vi "Get Section Indentation Length.vi"(10 "sections":string[](array[string]), 11 "info data":string) -> (3 "Indentation length":i32)   [LabVIEW 2013, in "infolib.lvlib"]
doc: "Checks if sections structure exists, if so divides string before the end of least significant section."
uses:
  infolib.lvlib
  <vilib>/regexp/Match Regular Expression.xnode
panel:
  out "submatch 1":string
  out "regexp":string
  # "testing string: (put \"1\" and \"2\" into section names)"
  # "blfdablad\n#startsection:: 1\njfkdla\n#startsection:: 2\ngroup2group2\n\t  \t#endsection:: 2\njdfkls\n#endsection:: 1\njfdklajfkdl"
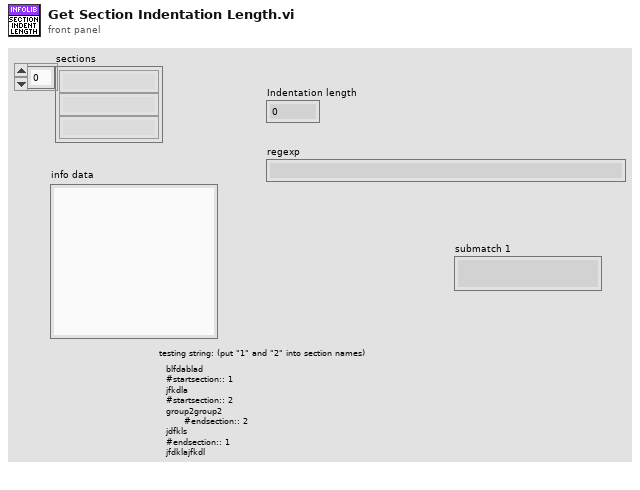
[diagram p1: front panel]
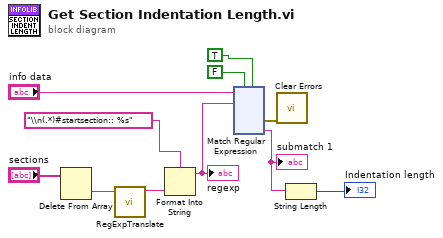
[diagram p0: block diagram]
diagram:
  n1 = Delete From Array(array="sections") -> (deleted portion=w2:string)  [unwired: 2 in, 1 out]
  n2 = call "RegExpTranslate.vi"("string"=w2) -> ("regexp safe string"=w1:string)  [unwired: 10 in]
  n3 = Format Into String(format string="\\n(.*)#startsection:: %s", w1) -> (resulting string=w6:string)  [unwired: 2 in, 1 out]
  "regexp" <- w6
  n4 = xnode "Match Regular Expression"("input string"="info data", "regular expression"=w6, "ignore case? (F)"=FALSE, "multiline? (F)"=TRUE) -> ("error out"=w5:errorcluster, "submatch 1"=w4:string)  [unwired: 2 in, 4 out]
  "submatch 1" <- w4
  n5 = call <vilib>:"Clear Errors.vi"("error in (no error)"=w5) -> ()  [unwired: 6 in, 1 out]
  n6 = String Length(string=w4) -> (length=→"Indentation length":i32)
